vi "PWM Heater.vi"() -> ()   [LabVIEW 2015]
uses:
  <vilib>/DAQmx/write.llb/DAQmx Write (Digital 1D Bool NChan 1Samp 1Line).vi
  <vilib>/DAQmx/miscellaneous.llb/DAQmx Fill In Error Info.vi
panel:
  in  "Cycle time (s)":dbl=5.0
  in  "Steps in a cycle":i32=256
  in  "stop":bool
  in  "Duty cycle % (0-100)":dbl=50.0
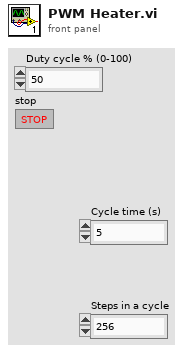
[diagram p1: front panel]
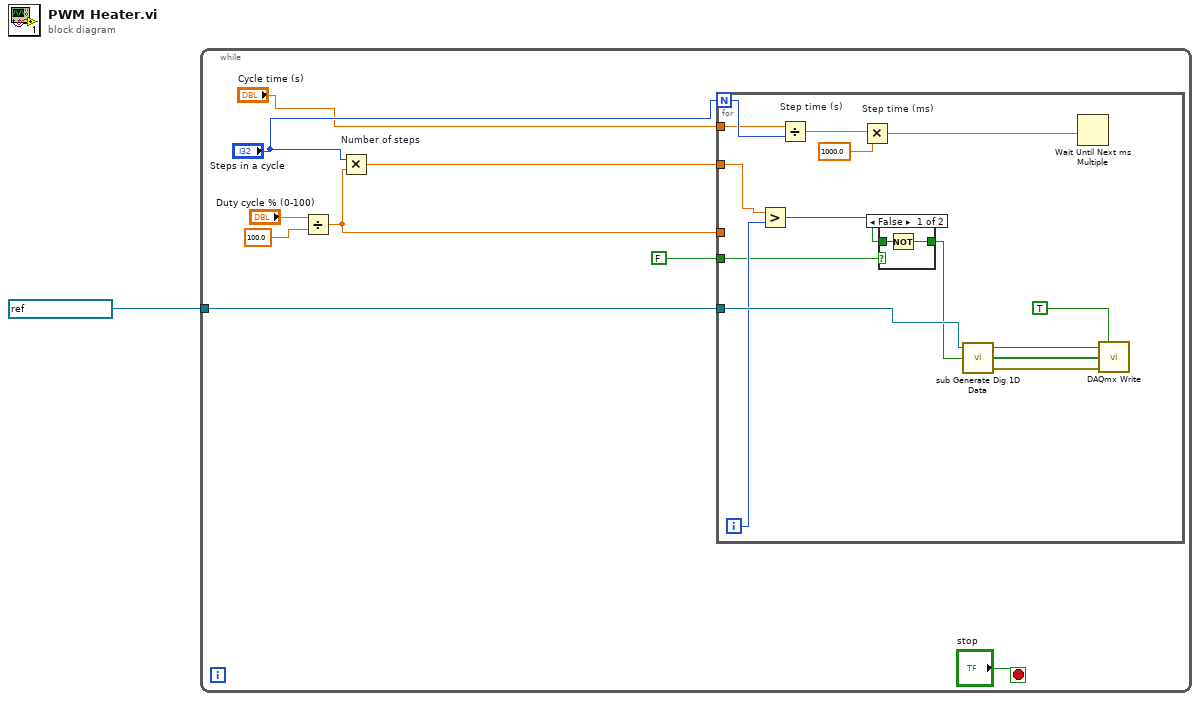
[diagram p0: block diagram]
diagram:
  n1 = while {
    tunnel: refnum<k21> "YellowdigOUT" -> [w10]
    stop <- "stop" stop-if-true
    n2 = Divide(x="Duty cycle % (0-100)", y=100.0) -> (x/y=w6:dbl)
    n3 = Multiply "Number of steps"(x="Steps in a cycle", y=w6) -> (x*y=w3:dbl)
    n4 = for {
      N: "Steps in a cycle" -> [w19]
      tunnel: w10 -> [w21]
      tunnel: w6 -> [_]
      tunnel: "Cycle time (s)" -> [w18]
      tunnel: w3 -> [w14]
      tunnel: FALSE -> [w11]
      i -> [w13]
      n5 = Greater?(x=w14, y=w13) -> (0:w12:bool)
      n6 = Divide "Step time (s)"(x=w18, y=w19) -> (x/y=w17:dbl)
      n7 = Multiply "Step time (ms)"(x=w17, y=1000.0) -> (x*y=w15:dbl)
      n8 = case shown="False" w11 {
        tunnel: [w26 w28] -> w20
        tunnel: w12 -> [w27 w28]
        frame False {
          n9 = Not(x=w27) -> (.not. x?=w26:bool)
        }
        frame True {
        }
      }
      n10 = call <vilib>:"sub Generate Dig 1D Data.vi"("initial value"=w20, "task in"=w21) -> ("error out"=w24:errorcluster, "Data"=w23:bool[], "task out"=w22:refnum<k21>)  [unwired: 1 in]
      n11 = Wait Until Next ms Multiple(millisecond multiple=w15) -> ()  [unwired: 1 out]
      n12 = call-poly <vilib>:"DAQmx Write.vi"("task/channels in"=w22, "auto start"=TRUE, "data"=w23, "error in"=w24) -> ()  [unwired: 9 in, 3 out]
    }
  }
